vi "Charts.vi"() -> ()   [LabVIEW 2013]
panel:
  out "System Temps":T1(graph)
  out "System Pressures":T2(graph)
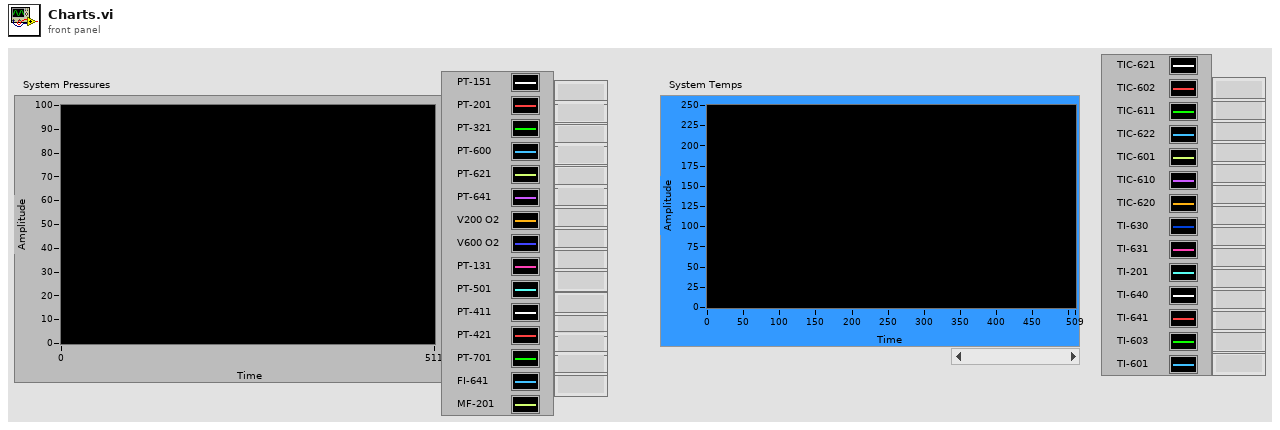
[diagram p1: front panel]
types:
  T1 = cluster{dbl, dbl, dbl, dbl, dbl, dbl, dbl, dbl, dbl, dbl, dbl, dbl, dbl, dbl}
  T2 = cluster{"Array of Double[0]":dbl, "Array of Double[1]":dbl, "Array of Double[2]":dbl, "Array of Double[3]":dbl, "Array of Double[4]":dbl, "Array of Double[5]":dbl, "Array of Double[6]":dbl, "Array of Double[7]":dbl, "Array of Double[8]":dbl, "Array of Double[9]":dbl, "Array of Double[10]":dbl, "Array of Double[11]":dbl, "Array of Double[12]":dbl, "Array of Double[13]":dbl, "Array of Double[14]":dbl}
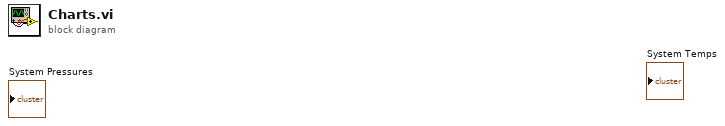
[diagram p0: block diagram]
diagram:
